vi "setHardCodedSettings.vi"(8 "error in (no error)":errorcluster, 11 "Electrometer in":refnum<class "Electrometer.lvclass">) -> (0 "error out":errorcluster, 3 "Electrometer out":refnum<class "Electrometer.lvclass">)   [LabVIEW 2016, in "Electrometer.lvclass"]
uses:
  Electrometer.lvclass
  TempUnits.ctl
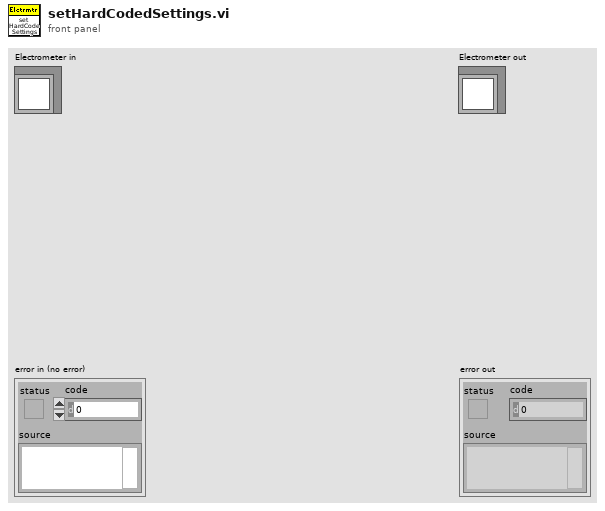
[diagram p1: front panel]
types:
  T1 = typedef "Electrometer.lvclass/TempUnits.ctl" = i32
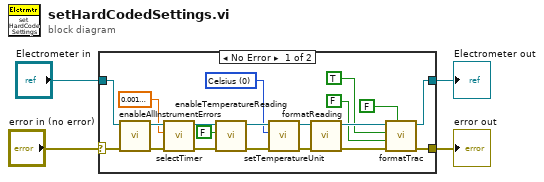
[diagram p0: block diagram]
diagram:
  n1 = case shown="No Error" "error in (no error)" {
    selector: "error in (no error)" -> [w19 w26]
    tunnel: [w10 w26] -> w3
    tunnel: [w11 w25] -> w1
    tunnel: "Electrometer in" -> [w18 w25]
    frame No Error {
      w20 = T1 0 items=["Celsius", "Fahrenheit", "Kelvin"] ("Temperature Unit (0: Celsius)")
      n2 = call "enableAllInstrumentErrors.vi"("error in (no error)"=w19, "Electrometer in"=w18) -> ("error out"=w17:errorcluster, "Electrometer out"=w16:refnum<class "Electrometer.lvclass">)  [unwired: 8 in]
      n3 = call "selectTimer.vi"("error in (no error)"=w17, "timer"=sgl 0.001, "Electrometer in"=w16) -> ("error out"=w14:errorcluster, "Electrometer out"=w15:refnum<class "Electrometer.lvclass">)  [unwired: 7 in]
      n4 = call "enableTemperatureReading.vi"("error in (no error)"=w14, "Enable Temperature (T: Enable)"=FALSE, "Electrometer in"=w15) -> ("error out"=w24:errorcluster, "Electrometer out"=w21:refnum<class "Electrometer.lvclass">)  [unwired: 7 in]
      n5 = call "setTemperatureUnit.vi"("error in (no error)"=w24, "Temperature Unit (0: Celsius)"=w20, "Electrometer in"=w21) -> ("error out"=w23:errorcluster, "Electrometer out"=w22:refnum<class "Electrometer.lvclass">)  [unwired: 7 in]
      n6 = call "formatReading.vi"("error in (no error)"=w23, "Electrometer in"=w22) -> ("error out"=w9:errorcluster, "Electrometer out"=w12:refnum<class "Electrometer.lvclass">)  [unwired: 8 in]
      n7 = call "formatTrac.vi"("Channel"=FALSE, "error in (no error)"=w9, "Temperature"=FALSE, "Timestamp"=TRUE, "Electrometer in"=w12) -> ("error out"=w10:errorcluster, "Electrometer out"=w11:refnum<class "Electrometer.lvclass">)  [unwired: 4 in, 1 out]
    }
    frame Error {
    }
  }
  "error out" <- w3
  "Electrometer out" <- w1
